vi "Save1_uc480.vi"(4 "Image filename save":string="D:\\Victor Sun\\optical trap control\\output_test\\test", 6 "save video?":bool, 7 "s32MemId":i32, 9 "save snapshot?":bool, 10 "Folder path save":path, 11 ".NET Refnum in":refnum<k24>) -> (3 "img saved to:":string)   [LabVIEW 2019]
doc: "Save snapshot or video (folder of images) from uc480/ThorCam DCx cameras"
uses:
  C:/Program Files/Thorlabs/Scientific Imaging/DCx Camera Support/Develop/DotNet/uc480DotNet.dll
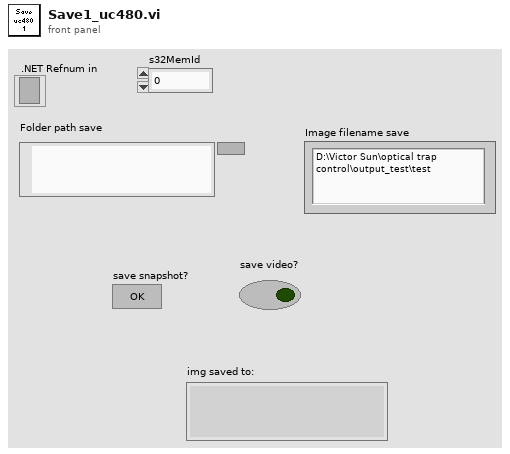
[diagram p1: front panel]
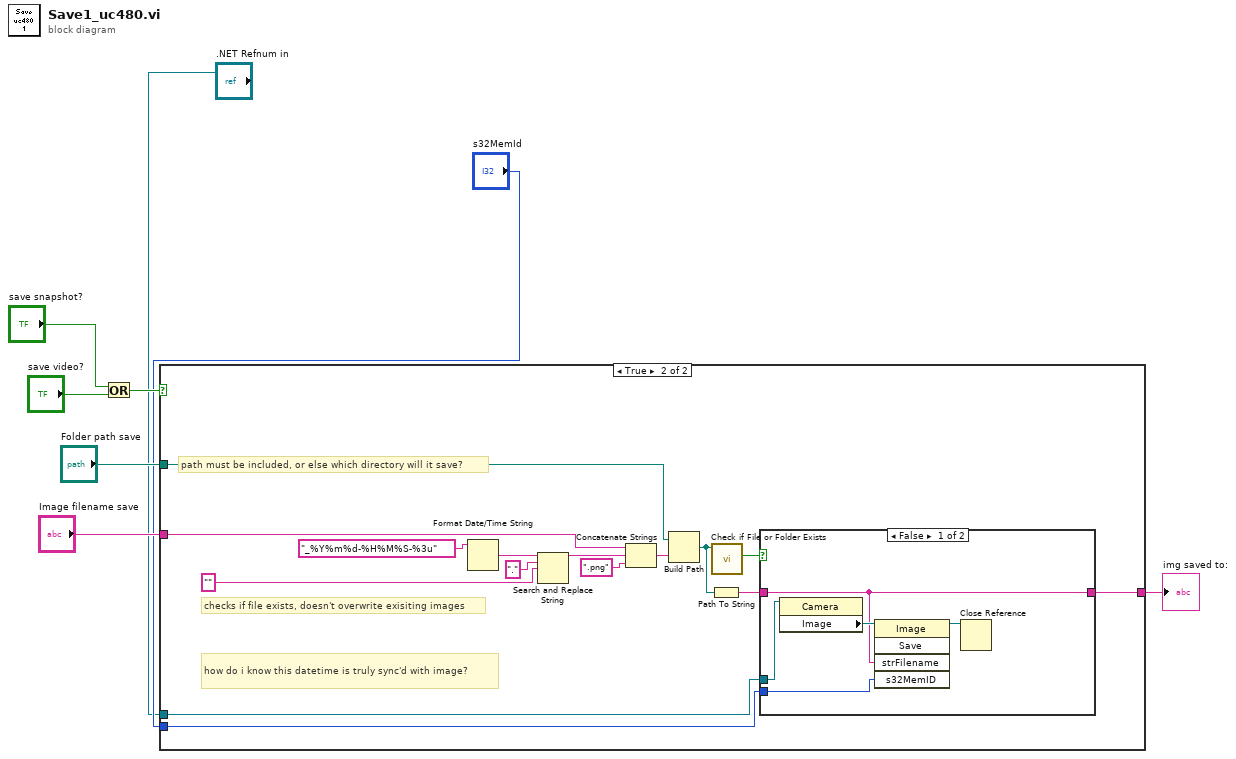
[diagram p0: block diagram]
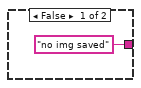
[diagram p2: hidden frame]
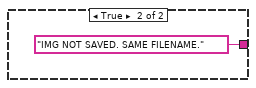
[diagram p3: hidden frame]
diagram:
  n1 = Or(x="save snapshot?", y="save video?") -> (x .or. y?=w6:bool)
  n2 = case shown="True" w6 {
    tunnel: ".NET Refnum in" -> [_ w24]
    tunnel: "s32MemId" -> [_ w23]
    tunnel: ["no img saved" ("snapshot filename") w19] -> w3
    tunnel: "Folder path save" -> [_ w11]
    tunnel: "Image filename save" -> [_ w10]
    frame False {
    }
    frame True {
      # "path must be included, or else which directory will it save?"
      # "checks if file exists, doesn't overwrite exisiting images"
      # "how do i know this datetime is truly sync'd with image?"
      n3 = Format Date/Time String(time format string (%c)="_%Y%m%d-%H%M%S-%3u") -> (date/time string=w18:string)  [unwired: 2 in]
      n4 = Search and Replace String(input string=w18, search string=".", replace string="" ("replace string (\"\")")) -> (result string=w14:string)  [unwired: 5 in, 3 out]
      n5 = Concatenate Strings(w10, w14, ".png" ("result string")) -> (w13:string)
      n6 = Build Path(base path=w11, name or relative path=w13) -> (appended path=w21:path)
      n7 = Path To String(path=w21) -> (string=w22:string)
      n8 = call <vilib>:"Check if File or Folder Exists.vi"("path"=w21) -> ("file or folder exists?"=w20:bool)  [unwired: 8 in, 2 out]
      n9 = case shown="False" w20 {
        tunnel: w24 -> [w27 _]
        tunnel: w23 -> [w26 _]
        tunnel: w22 -> [w25 _]
        tunnel: [w25 "IMG NOT SAVED. SAME FILENAME."] -> w19
        frame False {
          n10 = property class="Camera"(reference=w27) -> ("Image"=w29:refnum<k24>)  [unwired: 1 in, 2 out]
          n11 = invoke class="Image" method="Save"(reference=w29, "strFilename"=w25, "s32MemID"=w26) -> (reference out=w28:refnum<k24>)  [unwired: 2 in, 4 out]
          n12 = Close Reference(reference=w28) -> ()  [unwired: 1 in, 1 out]
        }
        frame True {
        }
      }
    }
  }
  "img saved to:" <- w3
